vi "Velocity Tracking.vi"() -> ()   [LabVIEW 2014]
uses:
  <vilib>/vision/NI_Vision_Development_Module.lvlib
panel:
  in  "Tab Control":enum32{"Analysis", "Plots"}(tab)
  in  "Average vessel diameter":dbl=30.0
  in  "Stop Button":bool
  in  "Calibration factor (1 pix = ? um)":dbl=1.45
  in  "X":dbl=323.0
  in  "Y":dbl=233.0
  in  "Correlation Index (0-1000)":dbl=600.0
  in  "Minimum Contrast":dbl=5.0
  in  "Search Window Width":dbl=65.0
  in  "Template Window Width":dbl=22.0
  in  "Search Window Seperation Height":dbl=10.0
  out "Matching":T1(plugin-control)
  in  "Stop Updating Panel":bool
  out "Particle Velocity - Unfiltered":dbl(graph)=nan
  out "selected path":path=path "C:/Users/Timothy/Desktop/020714 Rat 1/Videos/20140207124700.avi-Stabilized.avi-Rotated.avi"
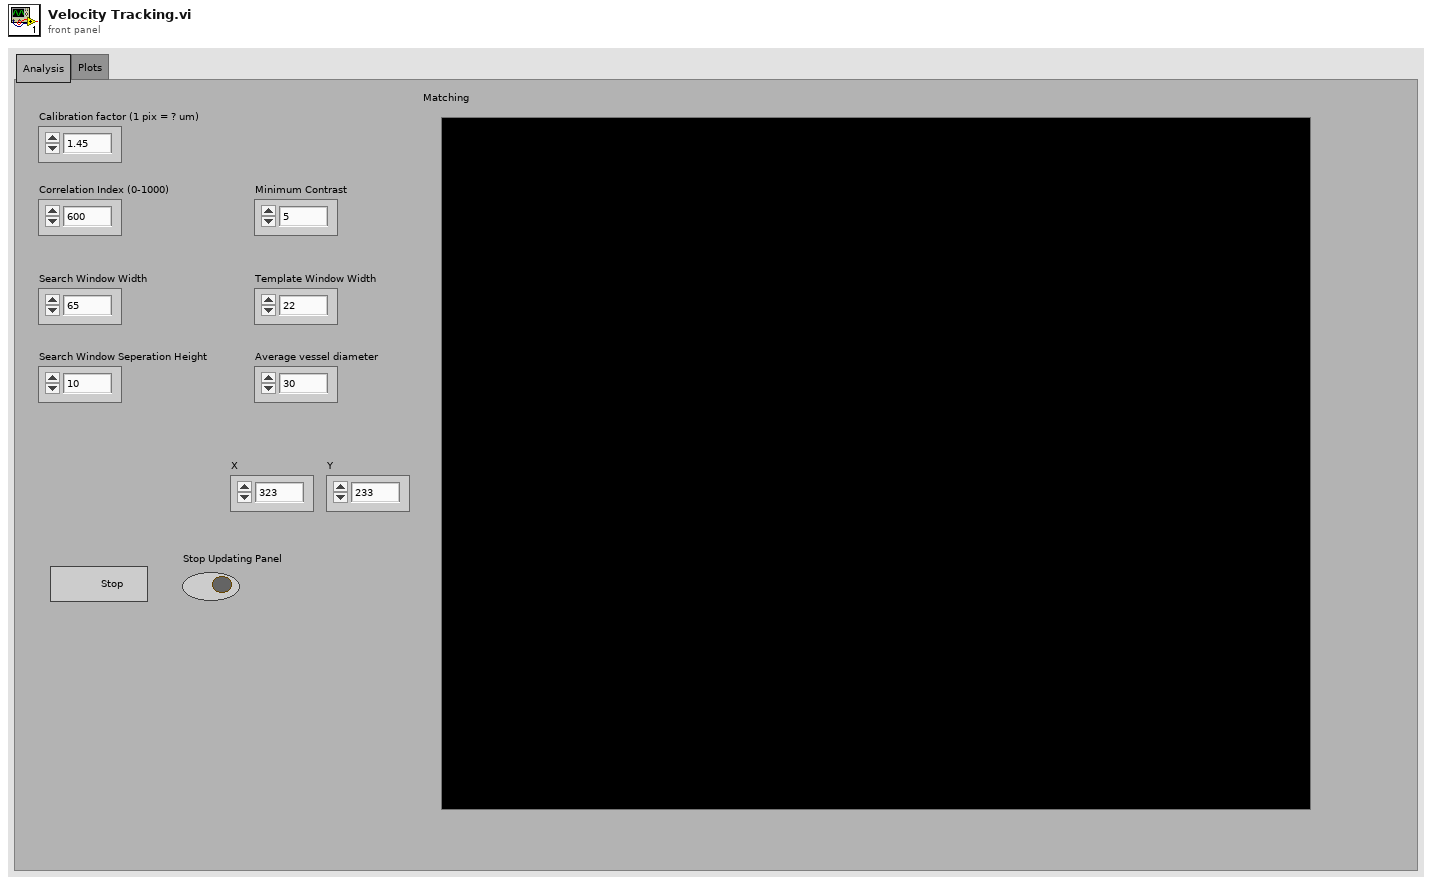
[diagram p1: front panel]
types:
  T1 = typedef "IMAQ Image.ctl" = refnum<image>
  T2 = typedef "AviRefnum.ctl" = refnum<k1>
  T3 = enum32{"AutoM", "Close", "Dilate", "Erode", "Gradient", "Gradient in", "Gradient out", "HitMiss", "Open", "PClose", "POpen", "Thick", "Thin"}
  T4 = typedef "ROI Descriptor" = cluster{"Global Rectangle":i32[], "Contours":cluster{"ID":enum32{"External", "Internal"}, "Type":u32, "Coordinates":i32[]}[]}
  T5 = cluster{"Position":cluster{"x":sgl, "y":sgl}, "Angle":sgl, "Scale":sgl, "Score":sgl, "Bounding Box":cluster{"x":sgl, "y":sgl}[]}[]
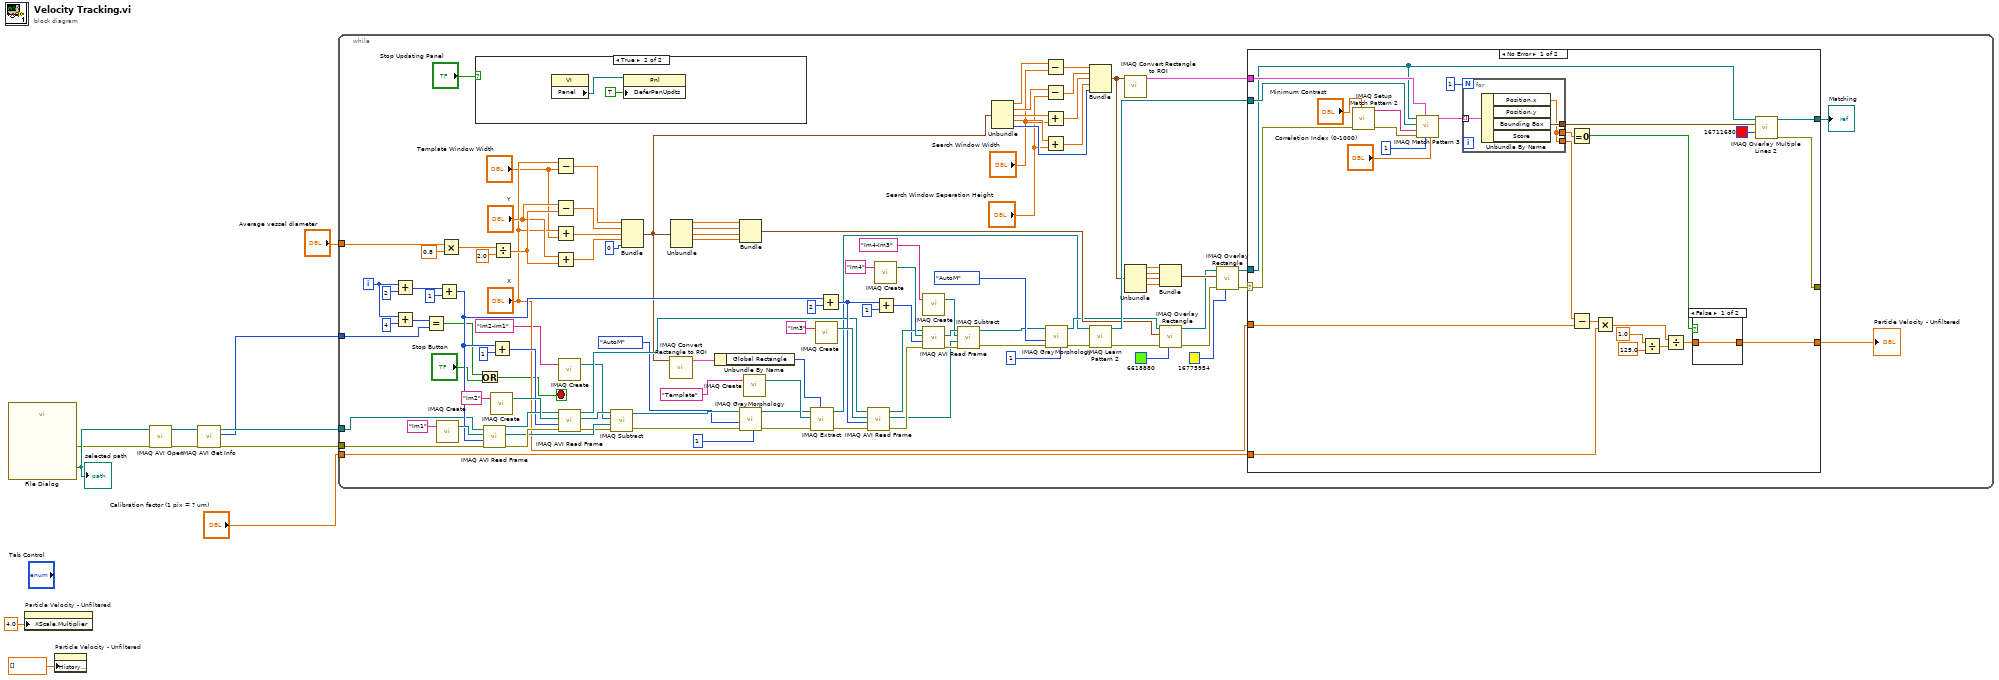
[diagram p0: block diagram]
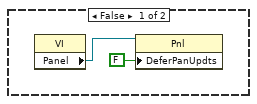
[diagram p2: hidden frame]
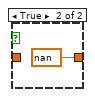
[diagram p3: hidden frame]
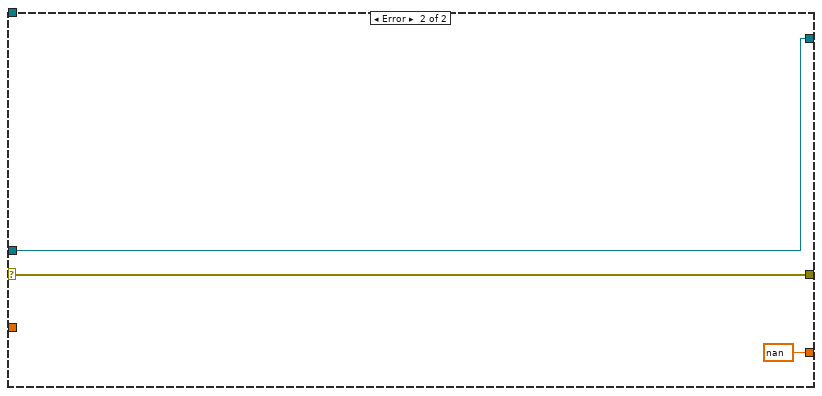
[diagram p4: hidden frame]
diagram:
  n1 = call "File Dialog"() -> ("selected path"=w8:path, "error out"=w7:errorcluster)  [unwired: 12 in, 2 out]
  "selected path" <- w8
  n2 = property on="Particle Velocity - Unfiltered" class="WFChart (strict)"("XScale.Multiplier"=4.0 ("X Scale.Offset and Multiplier:Multiplier")) -> ()  [unwired: 2 in, 2 out]
  n3 = property on="Particle Velocity - Unfiltered" class="WFChart (strict)"("History Data"=dbl[] []) -> ()  [unwired: 2 in, 2 out]
  n4 = call "IMAQ AVI Open"("error in (no error)"=w7, "AVI Path"=w8) -> ("error out"=w10:errorcluster, "Avi Refnum"=w11:T2)  [unwired: 8 in]
  n5 = call "IMAQ AVI Get Info"("error in (no error)"=w10, "Avi Refnum"=w11) -> ("error out"=w6:errorcluster, "Number of Frames"=w3:u32, "Avi Refnum (duplicate)"=w5:T2)  [unwired: 5 in, 2 out]
  n6 = while {
    tunnel: "Calibration factor (1 pix = ? um)" -> [w91]
    tunnel: "Average vessel diameter" -> [w12]
    tunnel: w6 -> [w59]
    tunnel: w5 -> [w58]
    tunnel: w3 -> [w38]
    i -> [w16]
    stop <- w23 stop-if-true
    n7 = Add(x=w16, y=2) -> (x+y=w14:i32)
    n8 = Add(x=w16, y=4) -> (x+y=w39:i32)
    n9 = Equal?(x=w39, y=w38) -> (x = y?=w24:bool)
    n10 = call "IMAQ Create"("Image Name"="Im1") -> ("New Image"=w112:T1)  [unwired: 4 in, 1 out]
    n11 = Add(x=w14, y=1) -> (x+y=w99:i32)
    n12 = Multiply(x=w12, y=0.8) -> (x*y=w84:dbl)
    n13 = case shown="True" "Stop Updating Panel" {
      frame False {
        n14 = property class="VI"() -> ("Panel"=w121:refnum<vi>)  [unwired: 2 in, 2 out]
        n15 = property class="Pnl"(reference=w121, "DeferPanUpdts"=FALSE ("Defer Panel Updates")) -> ()  [unwired: 1 in, 2 out]
      }
      frame True {
        n16 = property class="VI"() -> ("Panel"=w123:refnum<vi>)  [unwired: 2 in, 2 out]
        n17 = property class="Pnl"(reference=w123, "DeferPanUpdts"=TRUE ("Defer Panel Updates")) -> ()  [unwired: 1 in, 2 out]
      }
    }
    n18 = Or(x=w24, y="Stop Button") -> (x .or. y?=w23:bool)
    n19 = call "IMAQ AVI Read Frame"("error in (no error)"=w59, "Frame Number"=w99, "Image"=w112, "Avi Refnum"=w58) -> ("error out"=w116:errorcluster, "Image Out"=w108:T1, "Avi Refnum (duplicate)"=w110:T2)  [unwired: 4 in, 1 out]
    n20 = call "IMAQ Create"("Image Name"="Im2") -> ("New Image"=w111:T1)  [unwired: 4 in, 1 out]
    n21 = Add(x=w99, y=1) -> (x+y=w98:i32)
    n22 = Divide(x=w84, y=2.0) -> (x/y=w89:dbl)
    n23 = Subtract(x="X", y="Template Window Width") -> (x-y=w81:dbl)
    n24 = Subtract(x="Y", y=w89) -> (x-y=w86:dbl)
    n25 = Add(x="X", y="Template Window Width") -> (x+y=w82:dbl)
    n26 = Add(x="Y", y=w89) -> (x+y=w87:dbl)
    n27 = call "IMAQ Create"("Image Name"="Im2-Im1") -> ("New Image"=w20:T1)  [unwired: 4 in, 1 out]
    n28 = call "IMAQ AVI Read Frame"("error in (no error)"=w116, "Frame Number"=w98, "Image"=w111, "Avi Refnum"=w110) -> ("error out"=w102:errorcluster, "Image Out"=w109:T1, "Avi Refnum (duplicate)"=w94:T2)  [unwired: 4 in, 1 out]
    n29 = call "IMAQ Subtract"("Image Src A"=w109, "Image Dst"=w20, "Image Src B"=w108, "error in (no error)"=w102) -> ("Image Dst Out"=w45:T1, "error out"=w44:errorcluster)  [unwired: 3 in]
    n30 = Bundle(w81, w86, w82, w87, 0) -> (w60:cluster{dbl, dbl, dbl, dbl, i32})  [unwired: 1 in]
    n31 = call "IMAQ Convert Rectangle to ROI"("Rectangle"=w60) -> ("ROI Descriptor"=w79:T4)  [unwired: 8 in, 1 out]
    n32 = Unbundle(w60) -> (w77:dbl, w76:dbl, w75:dbl, w74:dbl)  [unwired: 1 out]
    n33 = Unbundle By Name(w79) -> ("Global Rectangle"=w78:i32[])
    n34 = call "IMAQ GrayMorphology"("Number of iterations (1)"=1, "error in (no error)"=w44, "Operation"=T3."AutoM", "Image Src"=w45) -> ("error out"=w34:errorcluster, "Image Dst Out"=w29:T1)  [unwired: 6 in]
    n35 = Bundle(w77, w76, w75, w74) -> (w53:cluster{dbl, dbl, dbl, dbl})  [unwired: 1 in]
    n36 = call "IMAQ Create"("Image Name"="Template") -> ("New Image"=w119:T1)  [unwired: 4 in, 1 out]
    n37 = call "IMAQ Extract"("Optional Rectangle"=w78, "error in (no error)"=w34, "Image Dst"=w119, "Image Src"=w29) -> ("error out"=w93:errorcluster, "Image Dst Out"=w27:T1)  [unwired: 6 in]
    n38 = call "IMAQ Create"("Image Name"="Im3") -> ("New Image"=w105:T1)  [unwired: 4 in, 1 out]
    n39 = Add(x=w99, y=2) -> (x+y=w96:i32)
    n40 = call "IMAQ AVI Read Frame"("error in (no error)"=w93, "Frame Number"=w96, "Image"=w105, "Avi Refnum"=w94) -> ("error out"=w115:errorcluster, "Image Out"=w21:T1, "Avi Refnum (duplicate)"=w103:T2)  [unwired: 4 in, 1 out]
    n41 = call "IMAQ Create"("Image Name"="Im4") -> ("New Image"=w104:T1)  [unwired: 4 in, 1 out]
    n42 = Add(x=w96, y=1) -> (x+y=w95:i32)
    n43 = call "IMAQ Create"("Image Name"="Im4-Im3") -> ("New Image"=w18:T1)  [unwired: 4 in, 1 out]
    n44 = call "IMAQ AVI Read Frame"("error in (no error)"=w115, "Frame Number"=w95, "Image"=w104, "Avi Refnum"=w103) -> ("error out"=w101:errorcluster, "Image Out"=w22:T1)  [unwired: 4 in, 2 out]
    n45 = call "IMAQ Subtract"("Image Src A"=w22, "Image Dst"=w18, "Image Src B"=w21, "error in (no error)"=w101) -> ("Image Dst Out"=w35:T1, "error out"=w43:errorcluster)  [unwired: 3 in]
    n46 = Unbundle(w60) -> (w62:dbl, w57:dbl, w56:dbl, w55:dbl, w69:i32)
    n47 = Subtract(x=w62, y="Search Window Width") -> (x-y=w73:dbl)
    n48 = Subtract(x=w57, y="Search Window Seperation Height") -> (x-y=w71:dbl)
    n49 = Add(x=w56, y="Search Window Width") -> (x+y=w72:dbl)
    n50 = Add(x=w55, y="Search Window Seperation Height") -> (x+y=w70:dbl)
    n51 = call "IMAQ GrayMorphology"("Number of iterations (1)"=1, "error in (no error)"=w43, "Operation"=T3."AutoM", "Image Src"=w35) -> ("error out"=w33:errorcluster, "Image Dst Out"=w28:T1)  [unwired: 6 in]
    n52 = Bundle(w73, w71, w72, w70, w69) -> (w61:cluster{dbl, dbl, dbl, dbl, i32})  [unwired: 1 in]
    n53 = call "IMAQ Learn Pattern 2"("error in (no error)"=w33, "Image"=w27) -> ("error out"=w49:errorcluster, "Template Image Out"=w92:T1)  [unwired: 8 in]
    n54 = call "IMAQ Convert Rectangle to ROI"("Rectangle"=w61) -> ("ROI Descriptor"=w68:T4)  [unwired: 8 in, 1 out]
    n55 = Unbundle(w61) -> (w67:dbl, w66:dbl, w65:dbl, w64:dbl)  [unwired: 1 out]
    n56 = Bundle(w67, w66, w65, w64) -> (w51:cluster{dbl, dbl, dbl, dbl})  [unwired: 1 in]
    n57 = call "IMAQ Overlay Rectangle"("Color"=u32 6618880, "error in (no error)"=w49, "Rectangle"=w53, "Image"=w28) -> ("error out"=w48:errorcluster, "Image Out"=w50:T1)  [unwired: 6 in]
    n58 = call "IMAQ Overlay Rectangle"("Color"=u32 16775954, "error in (no error)"=w48, "Rectangle"=w51, "Image"=w50) -> ("error out"=w47:errorcluster, "Image Out"=w46:T1)  [unwired: 6 in]
    n59 = case shown="No Error" w47 {
      selector: w47 -> [w151 w159]
      tunnel: w92 -> [w149 _]
      tunnel: w91 -> [w145 _]
      tunnel: [w138 w158] -> w90
      tunnel: [w139 w159] -> _
      tunnel: w68 -> [w144 _]
      tunnel: "X" -> [w131 _]
      tunnel: w46 -> [w137 w158]
      tunnel: [w134 nan] -> w26
      frame No Error {
        n60 = call "IMAQ Setup Match Pattern 2"("Minimum Contrast"="Minimum Contrast", "error in (no error)"=w151) -> ("error out"=w142:errorcluster, "Match Pattern Setup Data"=w143:string)  [unwired: 8 in]
        n61 = call "IMAQ Match Pattern 3"("Minimum Match Score"="Correlation Index (0-1000)", "Number of Matches Requested"=1, "ROI Descriptor"=w144, "error in (no error)"=w142, "Match Pattern Setup Data"=w143, "Template Image"=w149, "Image"=w137) -> ("Matches"=w147:T5)  [unwired: 2 in, 2 out]
        n62 = for {
          N: 1 -> [_]
          tunnel: [w156] -> w141
          tunnel: [w154] -> w130
          tunnel: w147 -> [w155] mode=indexing
          tunnel: [w154] -> w135
          n63 = Unbundle By Name(w155) -> ("Position.x"=w154:sgl, "Bounding Box"=w156:cluster{"x":sgl, "y":sgl}[])  [unwired: 2 out]
        }
        n64 = Equal To 0?(x=w135) -> (x = 0?=w136:bool)
        n65 = Subtract(x=w130, y=w131) -> (x-y=w146:dbl)
        n66 = Multiply(x=w146, y=w145) -> (x*y=w126:dbl)
        n67 = Divide(x=1.0, y=125.0) -> (x/y=w127:dbl)
        n68 = Divide(x=w126, y=w127) -> (x/y=w125:dbl)
        n69 = case shown="False" w136 {
          tunnel: [w152 nan] -> w134
          tunnel: w125 -> [w152 _]
          frame False {
          }
          frame True {
          }
        }
        n70 = call "IMAQ Overlay Multiple Lines 2"("Image"=w137, "Line End Points"=w141, "Color"=u32 16711680) -> ("Image Out"=w138:T1, "error out"=w139:errorcluster)  [unwired: 11 in]
      }
      frame Error {
      }
    }
    "Matching" <- w90
    "Particle Velocity - Unfiltered" <- w26
  }
